vi "IV to tsv.vi"(8 "experiment name":string, 9 "Iteration":i32, 10 "Sweep parameters":T1, 11 "Output IV":cluster{dbl[], dbl[]}) -> ()   [LabVIEW 2016]
uses:
  <vilib>/MakerHub/Toolbox/LMH-Toolbox.lvlib
panel:
  out "appended path":path
  out "appended array":dbl[][](array[numeric])
  out "spreadsheet string":string
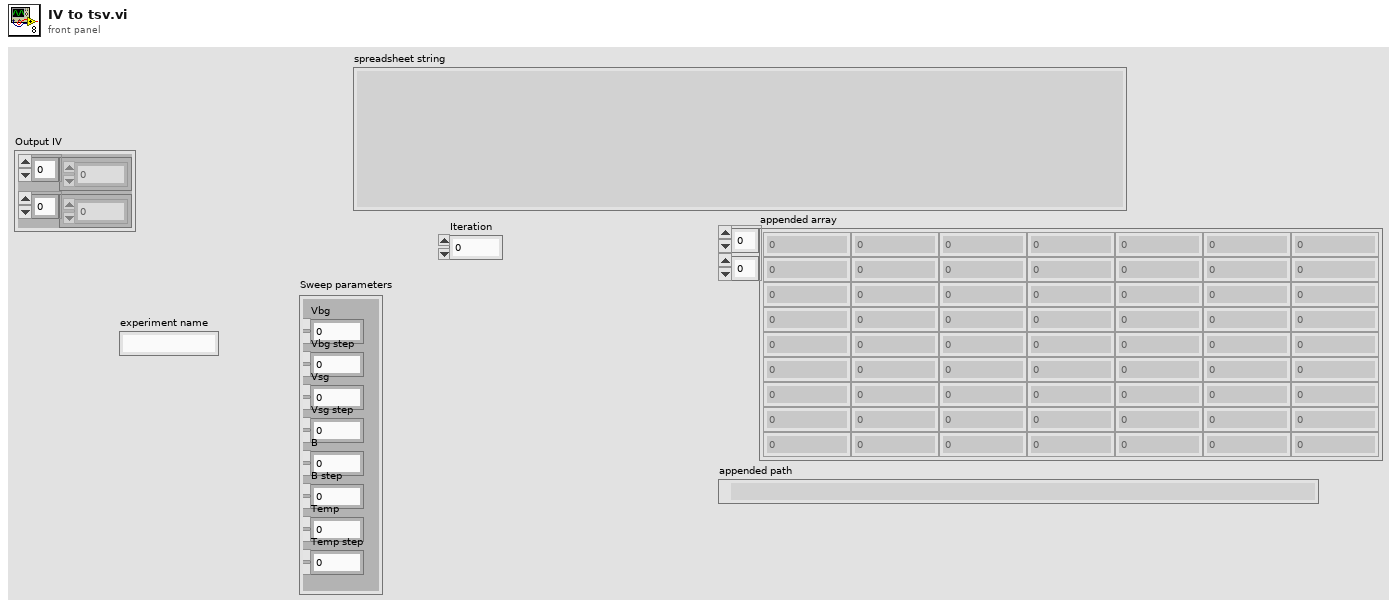
[diagram p1: front panel]
types:
  T1 = cluster{"Vbg":dbl, "Vbg step":dbl, "Vsg":dbl, "Vsg step":dbl, "B":dbl, "B step":dbl, "Temp":dbl, "Temp step":dbl}
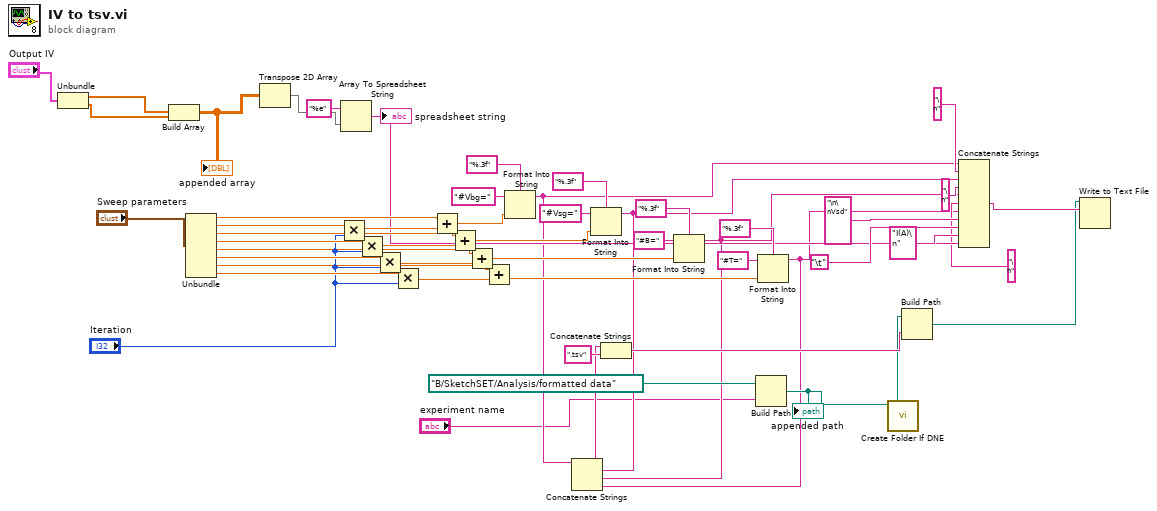
[diagram p0: block diagram]
diagram:
  n1 = Unbundle("Output IV") -> (w51:dbl[], w50:dbl[])
  n2 = Build Array(w51, w50) -> (w35:dbl[][])
  "appended array" <- w35
  n3 = Unbundle("Sweep parameters") -> ("Vbg"=w44:dbl, "Vbg step"=w48:dbl, "Vsg"=w42:dbl, "Vsg step"=w47:dbl, "B"=w40:dbl, "B step"=w46:dbl, "Temp"=w38:dbl, "Temp step"=w45:dbl)
  n4 = Transpose 2D Array(2D array=w35) -> (transposed array=w34:dbl[][])
  n5 = Multiply(x=w48, y="Iteration") -> (x*y=w43:dbl)
  n6 = Array To Spreadsheet String(array=w34, 3:"%e" ("format string")) -> (spreadsheet string=w20:string)  [unwired: 1 in]
  "spreadsheet string" <- w20
  n7 = Multiply(x=w47, y="Iteration") -> (x*y=w41:dbl)
  n8 = Multiply(x=w46, y="Iteration") -> (x*y=w39:dbl)
  n9 = Multiply(x=w45, y="Iteration") -> (x*y=w37:dbl)
  n10 = Add(x=w44, y=w43) -> (x+y=w33:dbl)
  n11 = Add(x=w42, y=w41) -> (x+y=w26:dbl)
  n12 = Add(x=w40, y=w39) -> (x+y=w25:dbl)
  n13 = Add(x=w38, y=w37) -> (x+y=w24:dbl)
  n14 = Format Into String(format string="%.3f", initial string="#Vbg=", w33) -> (resulting string=w8:string)  [unwired: 1 in, 1 out]
  n15 = Format Into String(format string="%.3f", initial string="#Vsg=", w26) -> (resulting string=w7:string)  [unwired: 1 in, 1 out]
  n16 = Format Into String(format string="%.3f", initial string="#B=", w25) -> (resulting string=w6:string)  [unwired: 1 in, 1 out]
  n17 = Build Path(base path=path "B:/SketchSET/Analysis/formatted data", name or relative path="experiment name") -> (appended path=w13:path)
  "appended path" <- w13
  n18 = Format Into String(format string="%.3f", initial string="#T=", w24) -> (resulting string=w5:string)  [unwired: 1 in, 1 out]
  n19 = Concatenate Strings(w8, w7, w6, w5) -> (w4:string)
  n20 = Concatenate Strings(w4, ".tsv" ("string")) -> (w15:string)
  n21 = call <vilib>:"Create Folder If DNE.vi"("Folder Path"=w13) -> ("Dup Path"=w12:path)  [unwired: 9 in, 1 out]
  n22 = Build Path(base path=w12, name or relative path=w15) -> (appended path=w17:path)
  n23 = Concatenate Strings(w8, "\n" ("string"), w7, "\n" ("string"), w6, "\n" ("string"), w5, "\n\nVsd" ("string"), "\t", "I(A)\n" ("string"), w20) -> (w19:string)
  n24 = Write to Text File(file (use dialog)=w17, text=w19) -> ()  [unwired: 2 in, 3 out]
